vi "Save Settings to XML.vi"(8 "error in (no error)":errorcluster, 11 "Settings":T1) -> (0 "error out":errorcluster)   [LabVIEW 2018, in "Settings Editor.lvlib"]
doc: "Saves the \"User Specified\" configuration data to an XML file. This is used to remember the users settings between executions.\n_____\nBased on Delacor QMH Project Template 4.1.0.59."
uses:
  Settings Editor.lvlib
  Settings--cluster.ctl
  Delacor/PPLs/CML_Shared.lvlibp/Signal Type--enum.ctl
  Delacor/PPLs/CML_Shared.lvlibp/Calibration Values--cluster.ctl
  <vilib>/Utility/xml.llb/Write to XML File(string).vi
  Delacor/PPLs/CML_Shared.lvlibp
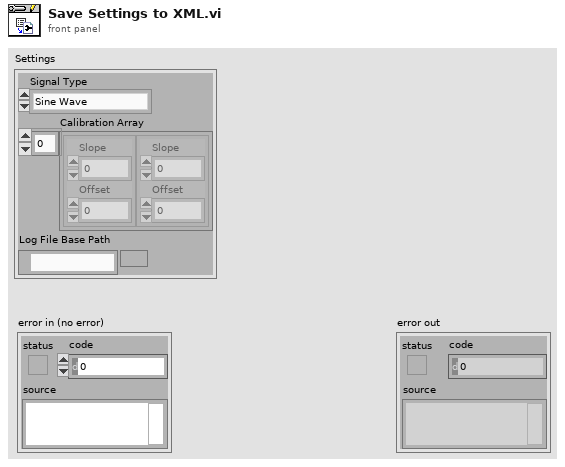
[diagram p1: front panel]
types:
  T1 = typedef "Settings Editor.lvlib/Settings--cluster.ctl" = cluster{"Signal Type":T2, "Calibration Array":T3[], "Log File Base Path":path}
  T2 = typedef "CML_Shared.lvlibp/Signal Type--enum.ctl" = enum16{"Sine Wave", "Square with Noise"}
  T3 = typedef "CML_Shared.lvlibp/Calibration Values--cluster.ctl" = cluster{"Slope":dbl, "Offset":dbl}
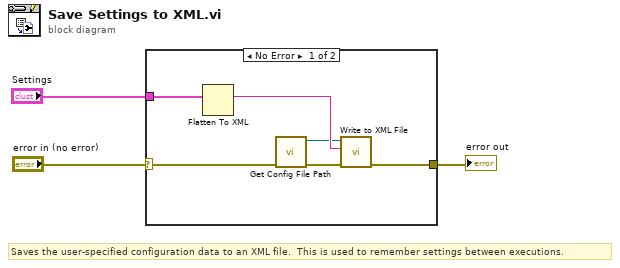
[diagram p0: block diagram]
diagram:
  # "Saves the user-specified configuration data to an XML file.  This is used to remember settings between executions."
  n1 = case shown="No Error" "error in (no error)" {
    selector: "error in (no error)" -> [w5 w10]
    tunnel: [w7 w10] -> w2
    tunnel: "Settings" -> [w9 _]
    frame No Error {
      n2 = Flatten To XML(anything=w9) -> (xml string=w8:string)
      n3 = call "Get Config File Path.vi"("error in (no error)"=w5) -> ("error out"=w4:errorcluster, "XML File Path"=w6:path)  [unwired: 9 in]
      n4 = call-poly <vilib>:"Write to XML File.vi"("error in (no error)"=w4, "XML Input"=w8, "XML File Path"=w6) -> ("error out"=w7:errorcluster)  [unwired: 6 in, 2 out]
    }
    frame Error {
    }
  }
  "error out" <- w2
